vi "icListen 1 Serial Number.vi"() -> ()   [LabVIEW 2020, in "PAM Library.lvlib"]
uses:
  PAM Library.lvlib
panel:
  in  "icListen 1 Serial Number":u16=4
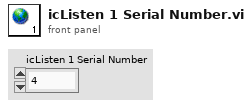
[diagram p1: front panel]
diagram:
